vi "facade.vi"(0 "Data In":T4, 2 "Display State In":T2, 3 "Container State":T3) -> (6 "Data Out":T4, 7 "Display State Out":T2, 8 "Action":T1)   [LabVIEW 2010, in "XUserDropdown.xctl"]
uses:
  XUserDropdown.xctl
  data.ctl
  <vilib>/_xctls/Container State.ctl
  state.ctl
  <vilib>/_xctls/Action.ctl
  global_variable.vi
  <vilib>/_xctls/XControlSupport.lvlib
panel:
  in  "user":string(combo)
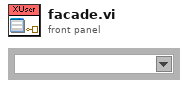
[diagram p1: front panel]
types:
  T1 = typedef "XControlSupport.lvlib/Action.ctl" = cluster{"Data Changed?":bool, "State Changed?":bool, "Action Name":string}
  T2 = typedef "XUserDropdown.xctl/state.ctl" = cluster{"error":errorcluster}
  T3 = typedef "XControlSupport.lvlib/Container State.ctl" = cluster{"Indicator?":bool, "Run Mode?":bool, " Refnum":refnum<vi>}
  T4 = typedef "XUserDropdown.xctl/data.ctl" = string
  T5 = enum8{"Enabled", "Disabled", "Disabled and Grayed Out"}
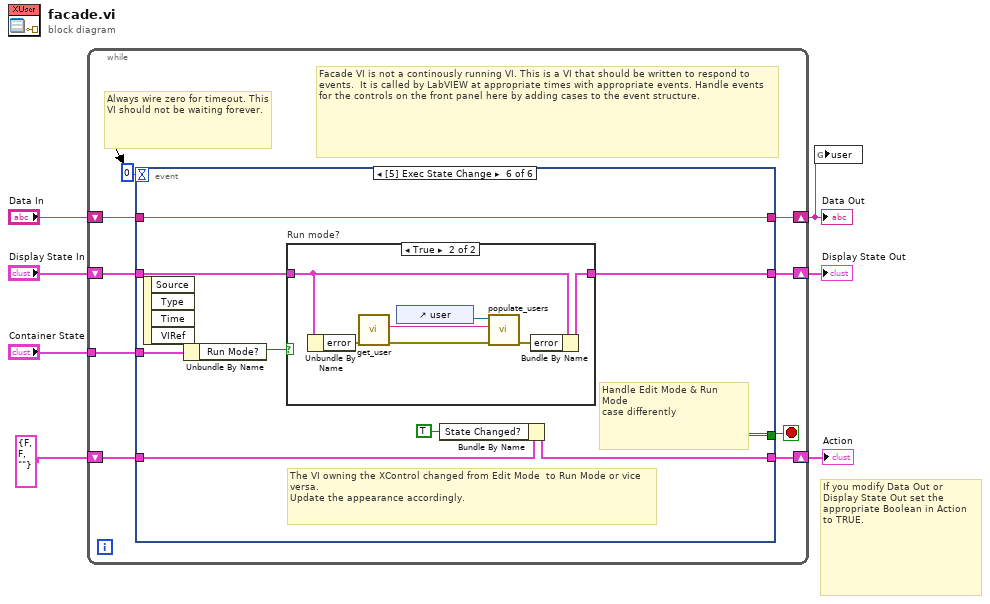
[diagram p0: block diagram]
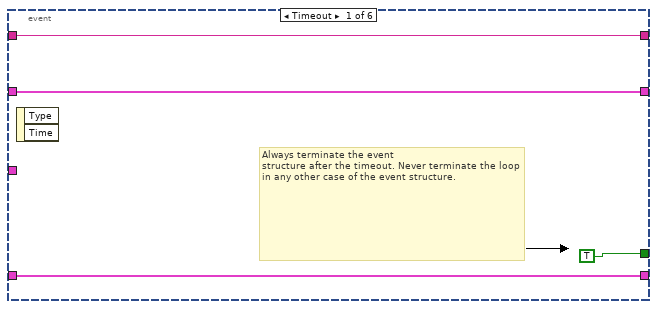
[diagram p2: hidden frame]
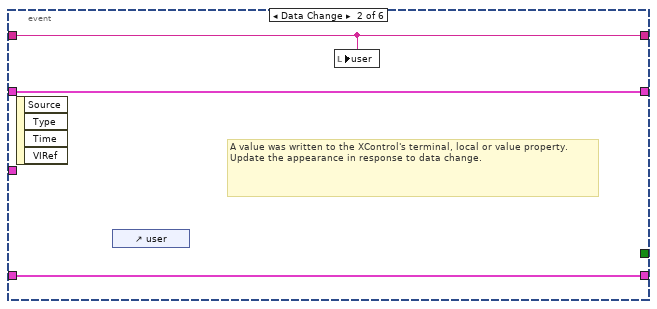
[diagram p3: hidden frame]
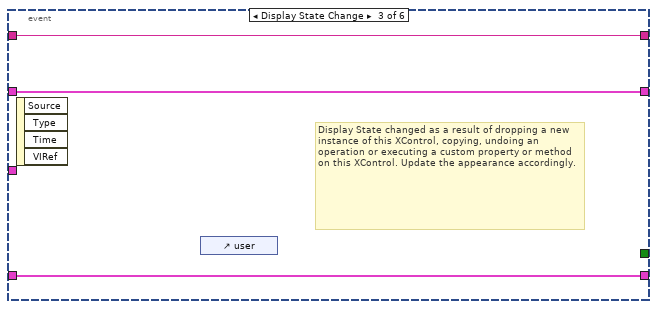
[diagram p4: hidden frame]
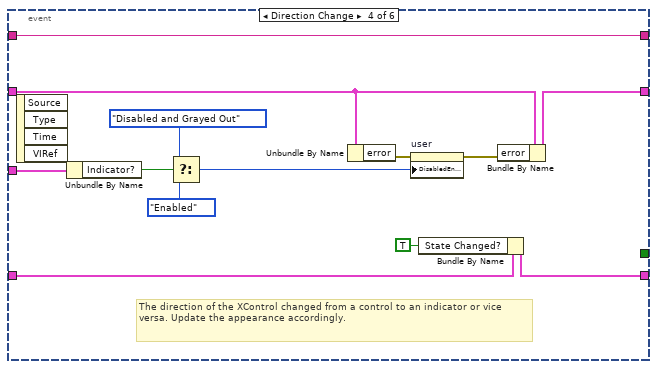
[diagram p5: hidden frame]
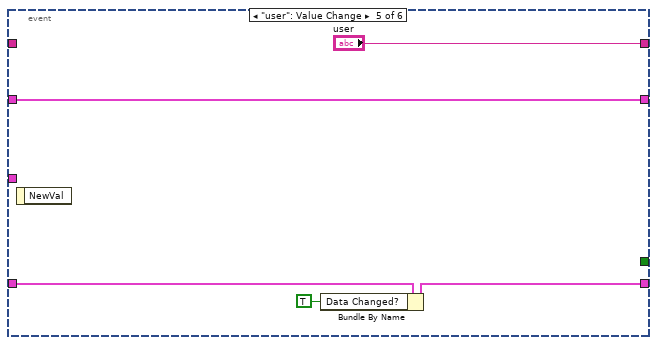
[diagram p6: hidden frame]
diagram:
  # "If you modify Data Out or\nDisplay State Out set the\nappropriate Boolean in Action\nto TRUE."
  n1 = while {
    shift-right: [w15] -> w5
    shift-left: "Display State In" -> [w16]
    tunnel: "Container State" -> [w12]
    shift-right: [w10] -> w1
    shift-left: "Data In" -> [w11]
    shift-right: [w8] -> w3
    shift-left: T1 {"Data Changed?"=FALSE, "State Changed?"=FALSE, "Action Name"=""} ("Action") -> [w9]
    stop <- w14 stop-if-true
    # "Facade VI is not a continously running VI. This is a VI that should be written to respond to events.  It is called by LabVIEW at appropriate times with appropriate events. Handle events for the controls on the front panel here by adding cases to the event structure."
    # "Always wire zero for timeout. This\nVI should not be waiting forever."
    n2 = event shown="[5] Exec State Change" {
      selector: _ -> [_ _ _ _ _ _]
      dyn-events: _ -> [_ _ _ _ _ _]
      timeout: 0 -> [_ _ _ _ _ _]
      tunnel: w16 -> [w18 w23 w26 w31 w43 w49]
      tunnel: [w18 w23 w26 w30 w43 w48] -> w15
      tunnel: [TRUE _ _ _ _ _] -> w14
      tunnel: w12 -> [_ _ _ w39 _ w52]
      tunnel: w11 -> [w17 w21 w24 w38 _ w51]
      tunnel: [w17 w21 w24 w38 "user" w51] -> w10
      tunnel: [w19 w22 w25 w27 w40 w45] -> w8
      tunnel: w9 -> [w19 w22 w25 w28 w41 w46]
      event Timeout {
        # "Always terminate the event\nstructure after the timeout. Never terminate the loop in any other case of the event structure."
        n3 = event-data() -> ()  [unwired: 1 in, 2 out]
      }
      event Data Change {
        # "A value was written to the XControl's terminal, local or value property.\nUpdate the appearance in response to data change."
        n4 = event-data() -> ()  [unwired: 1 in, 4 out]
        n5 = control-ref of="user"() -> ()  [unwired: 1 out]
        n6 = local write "user"(w21) -> ()
      }
      event Display State Change {
        # "Display State changed as a result of dropping a new instance of this XControl, copying, undoing an operation or executing a custom property or method on this XControl. Update the appearance accordingly."
        n7 = event-data() -> ()  [unwired: 1 in, 4 out]
        n8 = control-ref of="user"() -> ()  [unwired: 1 out]
      }
      event Direction Change {
        # "The direction of the XControl changed from a control to an indicator or vice versa. Update the appearance accordingly."
        n9 = event-data() -> ()  [unwired: 1 in, 4 out]
        n10 = Unbundle By Name(w39) -> ("Indicator?"=w37:bool)
        n11 = Select(t=T5."Disabled and Grayed Out" ("Disabled"), s=w37, f=T5."Enabled") -> (s? t:f=w35:T5)
        n12 = Unbundle By Name(w31) -> ("error"=w33:errorcluster)
        n13 = property on="user" class="CmbBox"(error in=w33, "DisabledEnum"=w35) -> (error out=w32:errorcluster)  [unwired: 1 in, 1 out]
        n14 = Bundle By Name(cluster=w28, "State Changed?"=TRUE ("Data Changed?")) -> (w27:T1)
        n15 = Bundle By Name(cluster=w31, "error"=w32) -> (w30:T2)
      }
      event "user": Value Change {
        n16 = event-data() -> ()  [unwired: 1 in, 1 out]
        n17 = Bundle By Name(cluster=w41, "Data Changed?"=TRUE) -> (w40:T1)
      }
      event Exec State Change {
        # "The VI owning the XControl changed from Edit Mode  to Run Mode or vice versa.\nUpdate the appearance accordingly."
        # "Handle Edit Mode & Run Mode\ncase differently"
        n18 = event-data() -> ()  [unwired: 1 in, 4 out]
        n19 = Unbundle By Name(w52) -> ("Run Mode?"=w50:bool)
        n20 = case "Run mode?" shown="True" w50 {
          tunnel: w49 -> [w53 w59]
          tunnel: [w53 w57] -> w48
          frame False {
          }
          frame True {
            n21 = Unbundle By Name(w59) -> ("error"=w56:errorcluster)
            n22 = call "get_user.vi"("error in (no error)"=w56) -> ("error out"=w55:errorcluster, "username out"=w54:string)  [unwired: 9 in]
            n23 = control-ref of="user"() -> (w60:refnum<vi>)
            n24 = call "populate_users.vi"("error in (no error)"=w55, "user name"=w54, "ref username in"=w60) -> ("error out"=w58:errorcluster)  [unwired: 7 in, 1 out]
            n25 = Bundle By Name(cluster=w59, "error"=w58) -> (w57:T2)
          }
        }
        n26 = Bundle By Name(cluster=w46, "State Changed?"=TRUE ("Data Changed?")) -> (w45:T1)
      }
    }
  }
  "Display State Out" <- w5
  "Data Out" <- w1
  "Action" <- w3
  n27 = global write "global_variable.vi" "user"(w1) -> ()
